vi "Position Calc_Build Reference Triangle_R1.vi"(0 "A2_in":sgl=81.899, 5 "A3_in":sgl=88.291, 9 "S1 (Length Between\n Cameras - inches)":sgl=2.25, 11 "Distance\nThreshold":sgl=500.0 format="%#_13g") -> (4 "S2":sgl, 6 "S3":sgl, 8 "Direction":i8=2, 10 "A2":sgl, 14 "A3":sgl, 15 "Accept":bool)   [LabVIEW 2015]
panel:
  out "Valid Angles":bool=TRUE
  in  "Backward - Upper Limit":sgl=350.0
  in  "Backward - Lower Limit":sgl=195.0
  in  "Forward - Upper Limit":sgl=165.0
  in  "Forward - Lower Limit":sgl=15.0
  out "Law of Sines\n Ratio":sgl=1.1133015e-05
  out "A1":sgl=6.3919983
  # "INTERMEDIATE VALUES"
  # "CALIBRATION/FILTERING"
  # "INPUTS"
  # "OUTPUTS"
  # "1 - Backwards (front toward beacon)\n2 - Forward (back toward beacon)"
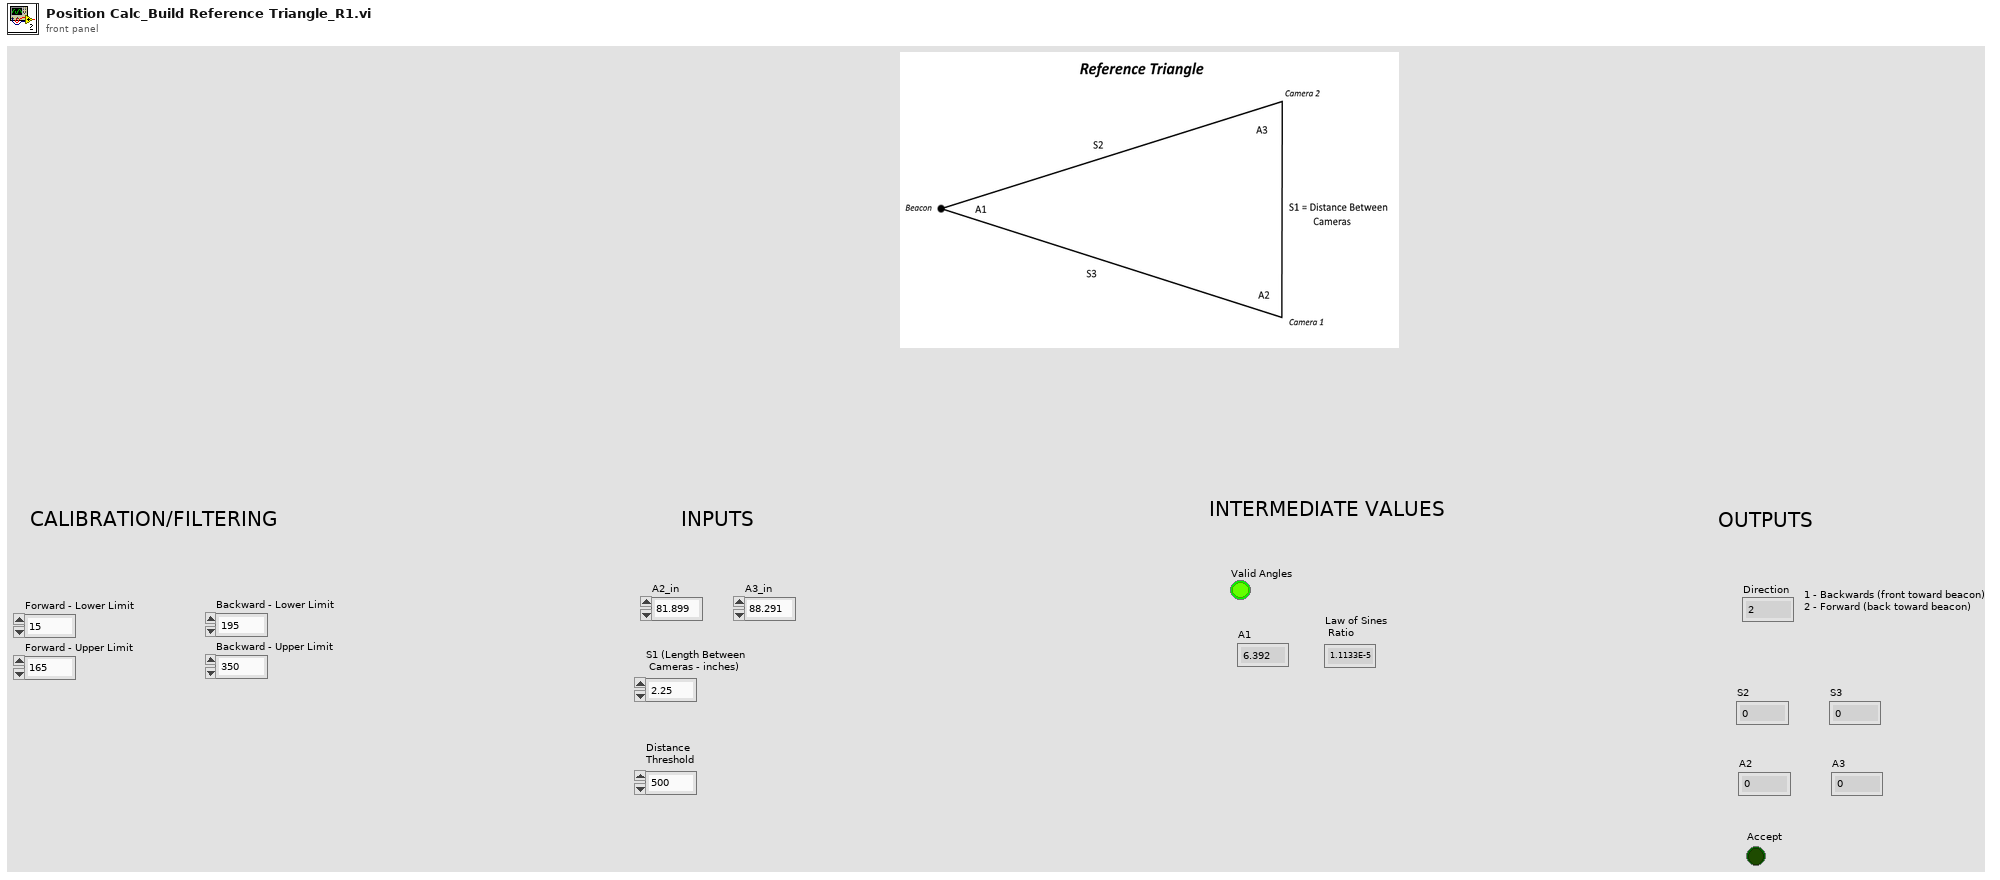
[diagram p1: front panel]
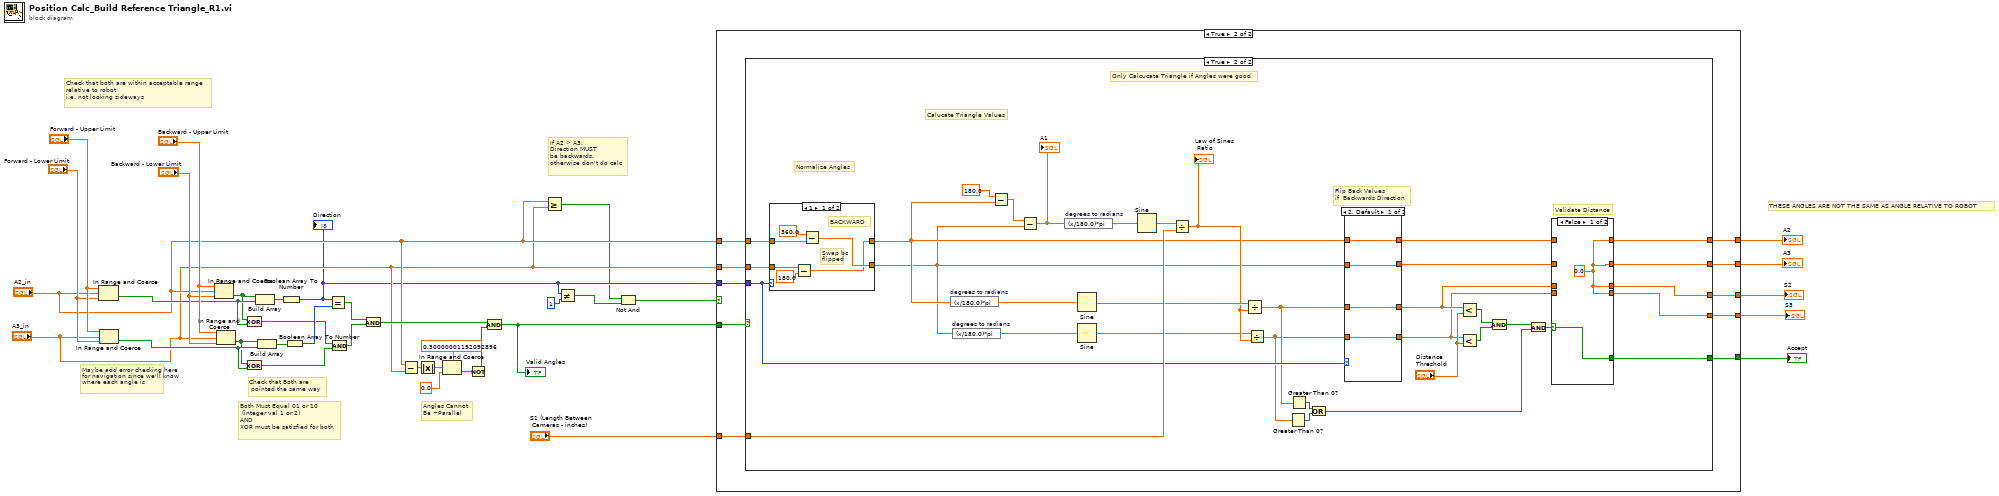
[diagram p0: block diagram]
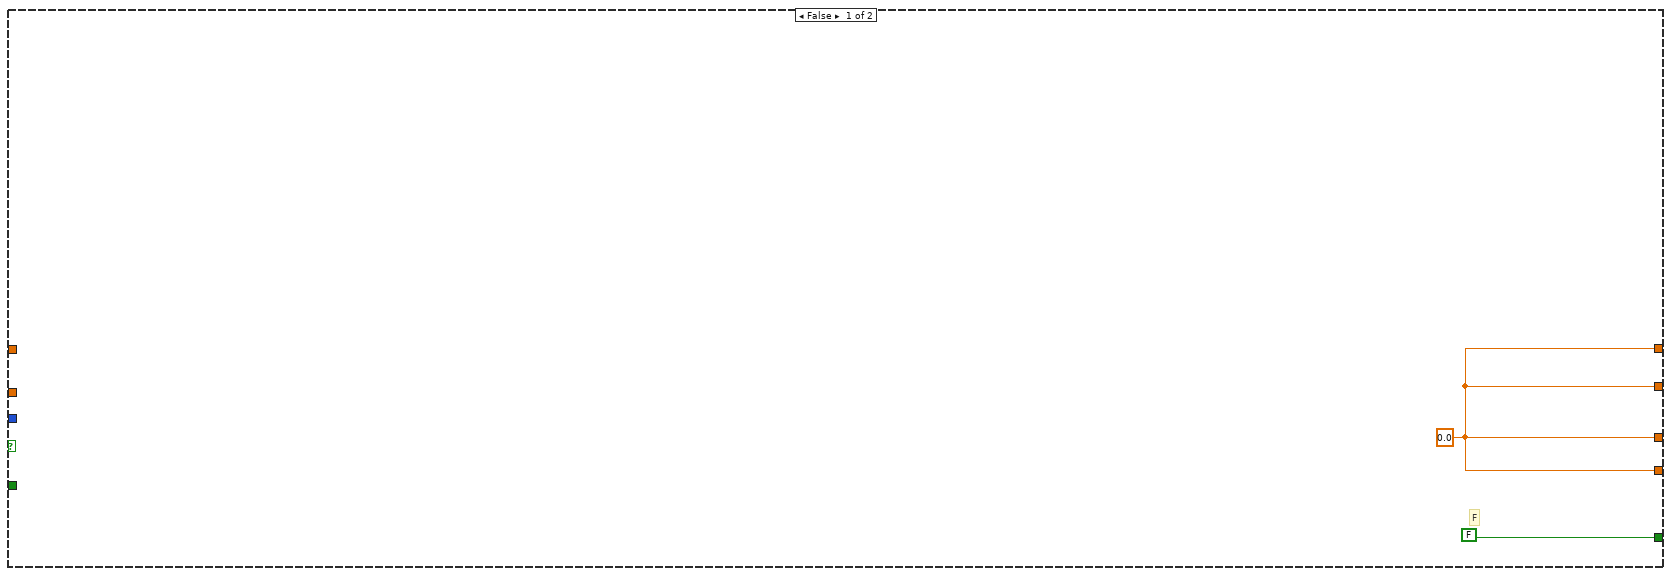
[diagram p2: hidden frame]
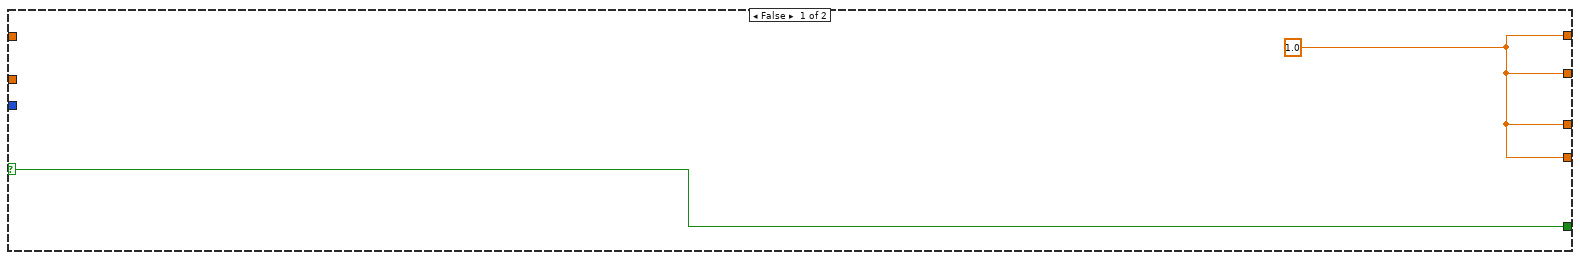
[diagram p3: hidden frame]
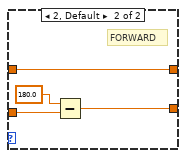
[diagram p6: hidden frame]
diagram:
  # "THESE ANGLES ARE NOT THE SAME AS ANGLE RELATIVE TO ROBOT"
  # "If A2 > A3,\nDirection MUST\nbe backwards,\notherwise don't do calc"
  # "Angles Cannot\nBe ~Parallel"
  # "Both Must Equal 01 or 10\n (integer val 1 or 2)\nAND\nXOR must be satisfied for both"
  # "Check that Both are\n pointed the same way"
  # "Maybe add error checking here \nfor navigation since we'll know \nwhere each angle is"
  # "Check that both are within acceptable range\nrelative to robot\ni.e. not looking sideways"
  n1 = In Range and Coerce(upper limit="Forward - Upper Limit", x="A2_in", lower limit="Forward - Lower Limit") -> (In Range?=w32:bool)  [unwired: 1 out]
  n2 = In Range and Coerce(upper limit="Forward - Upper Limit", x="A3_in", lower limit="Forward - Lower Limit") -> (In Range?=w30:bool)  [unwired: 1 out]
  n3 = In Range and Coerce(upper limit="Backward - Upper Limit", x="A2_in", lower limit="Backward - Lower Limit") -> (In Range?=w31:bool)  [unwired: 1 out]
  n4 = In Range and Coerce(upper limit="Backward - Upper Limit", x="A3_in", lower limit="Backward - Lower Limit") -> (In Range?=w29:bool)  [unwired: 1 out]
  n5 = Exclusive Or(1:w32, 2:w31) -> (0:w25:bool)
  n6 = Exclusive Or(1:w30, 2:w29) -> (0:w24:bool)
  n7 = Build Array(w31, w32) -> (w28:bool[])
  n8 = Build Array(w29, w30) -> (w27:bool[])
  n9 = Boolean Array To Number(Boolean array=w28) -> (number=w10:u32)
  "Direction" <- w10
  n10 = Boolean Array To Number(Boolean array=w27) -> (number=w26:u32)
  n11 = Equal?(x=w10, y=w26) -> (x = y?=w23:bool)
  n12 = And(x=w25, y=w24) -> (x .and. y?=w22:bool)
  n13 = And(x=w23, y=w22) -> (x .and. y?=w18:bool)
  n14 = Subtract(x="A2_in", y="A3_in") -> (x-y=w21:sgl)
  n15 = Absolute Value(x=w21) -> (abs(x)=w15:sgl)
  n16 = In Range and Coerce(upper limit=sgl 0.3, x=w15, lower limit=sgl 0.0) -> (In Range?=w14:bool)  [unwired: 1 out]
  n17 = Not(x=w14) -> (.not. x?=w16:bool)
  n18 = And(x=w18, y=w16) -> (x .and. y?=w17:bool)
  "Valid Angles" <- w17
  n19 = Greater Or Equal?(x="A2_in", y="A3_in") -> (x >= y?=w6:bool)
  n20 = Not Equal?(x=w10, y=1) -> (x != y?=w7:bool)
  n21 = Not And(1:w7, 2:w6) -> (0:w8:bool)
  n22 = case shown="True" w8 {
    tunnel: w10 -> [_ w48]
    tunnel: "A3_in" -> [_ w47]
    tunnel: w17 -> [_ w46]
    tunnel: "A2_in" -> [_ w45]
    tunnel: "S1 (Length Between\n Cameras - inches)" -> [_ w44]
    tunnel: [w38 w43] -> w5
    tunnel: [w38 w42] -> w4
    tunnel: [w38 w41] -> w3
    tunnel: [w38 w40] -> w2
    tunnel: [FALSE w39] -> w1
    frame False {
      w38 = sgl 0.0
      # "F"
    }
    frame True {
      n23 = case shown="True" w46 {
        selector: w46 -> [w49 _]
        tunnel: w48 -> [_ w72]
        tunnel: w45 -> [_ w85]
        tunnel: w47 -> [_ w84]
        tunnel: w44 -> [_ w78]
        tunnel: [w49 w51] -> w39
        tunnel: [w50 w64] -> w41
        tunnel: [w50 w63] -> w40
        tunnel: [w50 w61] -> w42
        tunnel: [w50 w59] -> w43
        frame False {
          w50 = sgl 1.0
        }
        frame True {
          # "Flip Back Values\nif  Backwards Direction"
          # "Validate Distance"
          # "Calucate Triangle Values"
          # "Normalize Angles"
          # "Only Calcucate Triangle if Angles were good"
          n24 = case shown="1" w72 {
            tunnel: w85 -> [w104 w107]
            tunnel: w84 -> [w103 w109]
            tunnel: [w102 w108] -> w70
            tunnel: [w101 w107] -> w71
            frame 1 {
              # "Swap bc\nflipped"
              # "BACKWARD"
              n25 = Subtract(x=w103, y=sgl 180.0) -> (x-y=w101:sgl)
              n26 = Subtract(x=sgl 360.0, y=w104) -> (x-y=w102:sgl)
            }
            frame 2, Default {
              # "FORWARD"
              n27 = Subtract(x=sgl 180.0, y=w109) -> (x-y=w108:sgl)
            }
          }
          n28 = expression code="(x/180.0)*pi" "degrees to radians"(w71) -> (w77:sgl)
          n29 = expression code="(x/180.0)*pi" "degrees to radians"(w70) -> (w76:sgl)
          n30 = Subtract(x=sgl 180.0, y=w71) -> (x-y=w82:sgl)
          n31 = Subtract(x=w82, y=w70) -> (x-y=w81:sgl)
          "A1" <- w81
          n32 = expression code="(x/180.0)*pi" "degrees to radians"(w81) -> (w80:sgl)
          n33 = Sine(x=w77) -> (sin(x)=w75:sgl)
          n34 = Sine(x=w76) -> (sin(x)=w73:sgl)
          n35 = Sine(x=w80) -> (sin(x)=w79:sgl)
          n36 = Divide(x=w79, y=w78) -> (x/y=w74:sgl)
          "Law of Sines\n Ratio" <- w74
          n37 = Divide(x=w75, y=w74) -> (x/y=w58:sgl)
          n38 = Divide(x=w73, y=w74) -> (x/y=w56:sgl)
          n39 = Greater Than 0?(x=w56) -> (x > 0?=w55:bool)
          n40 = Greater Than 0?(x=w58) -> (x > 0?=w57:bool)
          n41 = Or(x=w57, y=w55) -> (x .or. y?=w52:bool)
          n42 = case shown="2, Default" w72 {
            tunnel: w58 -> [w96 w100]
            tunnel: w56 -> [w95 w99]
            tunnel: [w95 w100] -> w65
            tunnel: [w96 w99] -> w66
            tunnel: w71 -> [w94 w98]
            tunnel: w70 -> [w93 w97]
            tunnel: [w93 w98] -> w62
            tunnel: [w94 w97] -> w60
            frame 2, Default {
            }
            frame 1 {
            }
          }
          n43 = Less?(x=w66, y="Distance\nThreshold") -> (x < y?=w68:bool)
          n44 = Less?(x=w65, y="Distance\nThreshold") -> (x < y?=w67:bool)
          n45 = And(x=w68, y=w67) -> (x .and. y?=w53:bool)
          n46 = And(x=w53, y=w52) -> (x .and. y?=w54:bool)
          n47 = case shown="False" w54 {
            selector: w54 -> [w87 w92]
            tunnel: [w87 w92] -> w51
            tunnel: w66 -> [_ w91]
            tunnel: [w86 w91] -> w64
            tunnel: w65 -> [_ w90]
            tunnel: [w86 w90] -> w63
            tunnel: [w86 w89] -> w61
            tunnel: w62 -> [_ w89]
            tunnel: w60 -> [_ w88]
            tunnel: [w86 w88] -> w59
            frame False {
              w86 = sgl 0.0
            }
            frame True {
            }
          }
        }
      }
    }
  }
  "Accept" <- w1
  "A2" <- w5
  "A3" <- w4
  "S3" <- w2
  "S2" <- w3
